vi "PR Set PRF.vi"(1 "PRF":i32) -> (0 "Success":bool)   [LabVIEW 2022 SP3, in "BS6006PRPLUS.lvlib"]
uses:
  BS6006PRPLUS.lvlib
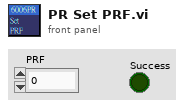
[diagram p1: front panel]
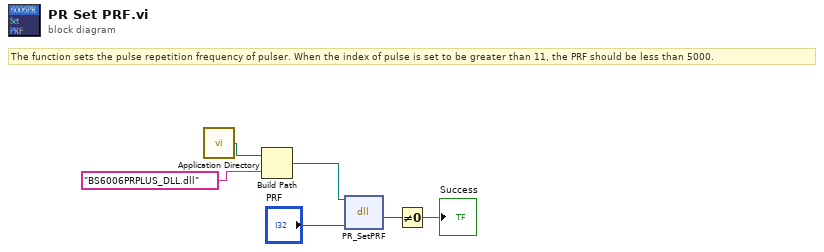
[diagram p0: block diagram]
diagram:
  # "The function sets the pulse repetition frequency of pulser. When the index of pulse is set to be greater than 11, the PRF should be less than 5000."
  n1 = call <vilib>:"Application Directory.vi"() -> ("Application Directory"=w3:path)
  n2 = Build Path(base path=w3, name or relative path="BS6006PRPLUS_DLL.dll") -> (appended path=w1:path)
  n3 = dll-call lib="E:/Broadsound_Program/PulserReceiver/6006PR PLUS/API/DLL/LabVIEW 15/VIs/BS6006PRPLUS_DLL.dll" fn="PR_SetPRF"(path in=w1, "PRF"="PRF") -> ("return type"=w5:u8)  [unwired: 3 in, 2 out]
  n4 = Not Equal To 0?(x=w5) -> (x != 0?=→"Success":bool)
